vi "Creator Queue.vi"(9 "Priority?":bool, 10 "Msg Strategy":refnum<class "Msg Strategy.lvclass">, 11 "qqqqq in":refnum<class "qqqqq.lvclass">) -> (3 "qqqqq out":refnum<class "qqqqq.lvclass">)   [LabVIEW 2021, in "Providers.lvlib" / "qqqqq.lvlib" / "qqqqq.lvclass"]
uses:
  jettl/Msg Strategy/Msg Strategy.lvclass
  qqqqq.lvclass
  qqqqq.lvclass/qqqqq.ctl
  jettl/Queue/Queue.lvclass
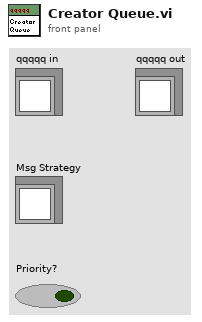
[diagram p1: front panel]
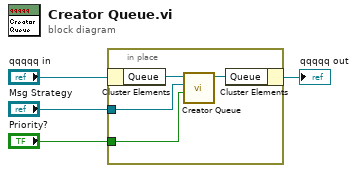
[diagram p0: block diagram]
diagram:
  n1 = in-place {
    in-place-border: "Msg Strategy" -> [w6]
    in-place-border: "Priority?" -> [w5]
    n2 = in-place-cluster #1("qqqqq in") -> ("Queue"=w8:refnum<class "Queue.lvclass">)
    n3 = call-dynamic "Creator Queue.vi"("Priority?"=w5, "Msg Strategy"=w6, "Queue in"=w8) -> ("Queue out"=w7:refnum<class "Queue.lvclass">)  [unwired: 8 in]
    n4 = in-place-cluster #1("Queue"=w7) -> (→"qqqqq out":refnum<class "qqqqq.lvclass">)
  }
